vi "uc480_SubVI_SetGain_JRtest.vi"(0 ".NET (Reference)":refnum<k24>, 5 "Gain":i32, 11 "Error In":errorcluster) -> (6 "Gain (out)":i32, 15 "Error Out":errorcluster)   [LabVIEW 2018]
uses:
  C:/Users/user/Desktop/Thorcam/uc480DotNet.dll
  uc480DotNet.dll
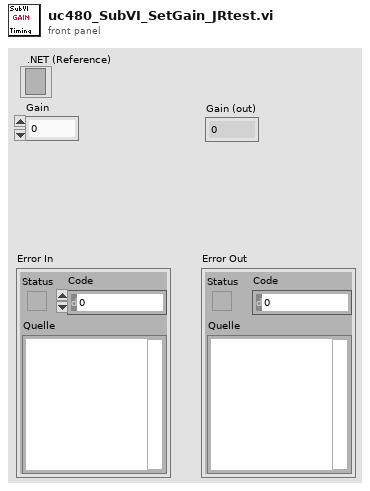
[diagram p1: front panel]
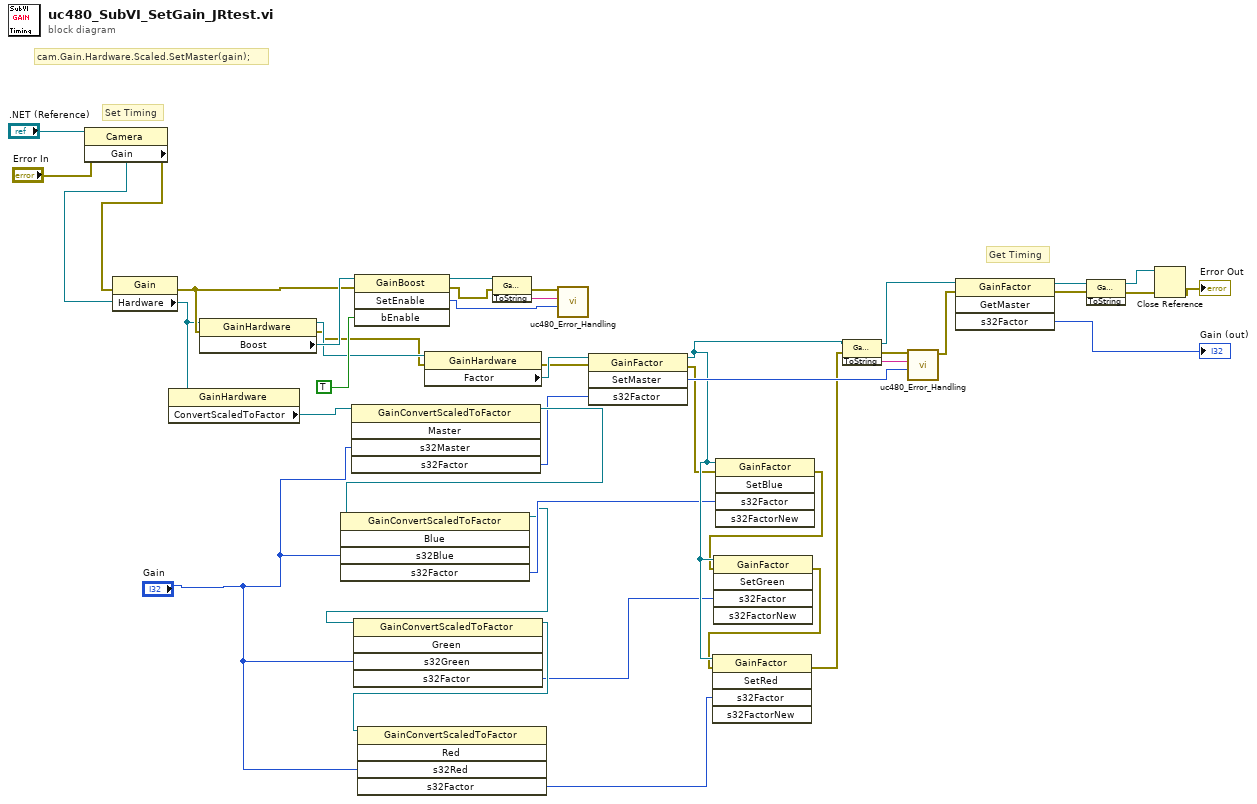
[diagram p0: block diagram]
diagram:
  # "cam.Gain.Hardware.Scaled.SetMaster(gain);"
  # "Get Timing"
  # "Set Timing"
  n1 = property class="Camera"(reference=".NET (Reference)", error in="Error In") -> (error out=w32:errorcluster, "Gain"=w39:refnum<k24>)  [unwired: 1 out]
  n2 = property class="Gain"(reference=w39, error in=w32) -> (error out=w18:errorcluster, "Hardware"=w14:refnum<k24>)  [unwired: 1 out]
  n3 = property class="GainHardware"(reference=w14) -> ("ConvertScaledToFactor"=w8:refnum<k24>)  [unwired: 1 in, 2 out]
  n4 = property class="GainHardware"(reference=w14, error in=w18) -> (reference out=w27:refnum<k24>, error out=w17:errorcluster, "Boost"=w31:refnum<k24>)
  n5 = invoke class="GainConvertScaledToFactor" method="Master"(reference=w8, "s32Master"="Gain") -> (reference out=w7:refnum<k24>, "s32Factor"=w5:i32)  [unwired: 3 in, 3 out]
  n6 = invoke class="GainConvertScaledToFactor" method="Blue"(reference=w7, "s32Blue"="Gain") -> (reference out=w12:refnum<k24>, "s32Factor"=w13:i32)  [unwired: 3 in, 3 out]
  n7 = invoke class="GainConvertScaledToFactor" method="Green"(reference=w12, "s32Green"="Gain") -> (reference out=w11:refnum<k24>, "s32Factor"=w10:i32)  [unwired: 3 in, 3 out]
  n8 = invoke class="GainBoost" method="SetEnable"(reference=w31, error in=w18, "bEnable"=TRUE) -> (reference out=w30:refnum<k24>, error out=w25:errorcluster, "SetEnable"=w16:i32)  [unwired: 1 in, 1 out]
  n9 = invoke class="GainConvertScaledToFactor" method="Red"(reference=w11, "s32Red"="Gain") -> ("s32Factor"=w9:i32)  [unwired: 3 in, 4 out]
  n10 = property class="GainHardware"(reference=w27, error in=w17) -> (error out=w24:errorcluster, "Factor"=w26:refnum<k24>)  [unwired: 1 out]
  n11 = invoke class="GainBoost" method="ToString"(reference=w30, error in=w25) -> (error out=w33:errorcluster, "ToString"=w40:string)  [unwired: 1 in, 1 out]
  n12 = call "uc480_Error_Handling.vi"("Error Code"=w16, "Error String"=w40, "Error In"=w33) -> ()  [unwired: 8 in, 1 out]
  n13 = invoke class="GainFactor" method="SetMaster"(reference=w26, error in=w24, "s32Factor"=w5) -> (reference out=w15:refnum<k24>, error out=w4:errorcluster, "SetMaster"=w21:i32)  [unwired: 1 in, 1 out]
  n14 = invoke class="GainFactor" method="SetBlue"(reference=w15, error in=w4, "s32Factor"=w13) -> (error out=w3:errorcluster)  [unwired: 2 in, 4 out]
  n15 = invoke class="GainFactor" method="SetGreen"(reference=w15, error in=w3, "s32Factor"=w10) -> (error out=w2:errorcluster)  [unwired: 2 in, 4 out]
  n16 = invoke class="GainFactor" method="SetRed"(reference=w15, error in=w2, "s32Factor"=w9) -> (error out=w1:errorcluster)  [unwired: 2 in, 4 out]
  n17 = invoke class="GainFactor" method="ToString"(reference=w15, error in=w1) -> (reference out=w19:refnum<k24>, error out=w22:errorcluster, "ToString"=w23:string)  [unwired: 1 in]
  n18 = call "uc480_Error_Handling.vi"("Error Code"=w21, "Error String"=w23, "Error In"=w22) -> ("Error Out"=w20:errorcluster)  [unwired: 8 in]
  n19 = invoke class="GainFactor" method="GetMaster"(reference=w19, error in=w20) -> (reference out=w37:refnum<k24>, error out=w36:errorcluster, "s32Factor"=→"Gain (out)":i32)  [unwired: 2 in, 1 out]
  n20 = invoke class="GainFactor" method="ToString"(reference=w37, error in=w36) -> (reference out=w34:refnum<k24>, error out=w35:errorcluster)  [unwired: 1 in, 1 out]
  n21 = Close Reference(reference=w34, error in (no error)=w35) -> (error out=→"Error Out":errorcluster)
